vi "Dialog - Add Control.vi"(7 "Control":T3 {"Mech.Action" items=["Switch when Pressed", "Switch when Released", "Switch until Released", "Latch when Pressed", "Latch when Released", "Latch until Released"]; "Type" items=["Numeric", "Spin Control", "Vertical Slide", "Horizontal Slide", "Push Button", "Rocker", "Vert Rocker", "Horizontal Toggle Switch", "Vertical Toggle Switch", "Slide Switch", "Vertical Slide Switch", "OK Button", "Square Push Button", "Round Push Button", "Vertical Slide Switch2", "Square Push Button2", "Round Push Button2", "Horizontal Slide Switch2", "Round LED", "Square LED"]}, 11 "error in (no error)":errorcluster) -> (8 "Control Out":T3 {"Mech.Action" items=["Switch when Pressed", "Switch when Released", "Switch until Released", "Latch when Pressed", "Latch when Released", "Latch until Released"]; "Type" items=["Numeric", "Spin Control", "Vertical Slide", "Horizontal Slide", "Push Button", "Rocker", "Vert Rocker", "Horizontal Toggle Switch", "Vertical Toggle Switch", "Slide Switch", "Vertical Slide Switch", "OK Button", "Square Push Button", "Round Push Button", "Vertical Slide Switch2", "Square Push Button2", "Round Push Button2", "Horizontal Slide Switch2", "Round LED", "Square LED"]}, 10 "Cancelled":bool, 15 "error out":errorcluster)   [LabVIEW 2011]
uses:
  Default.ctl
panel:
  in  "Switched when pressed":T1 {"HSlide" scale=0.0..10.0; "VSlide" scale=0.0..10.0; "Box" min=0.0 max=10.0}
  in  "Switched when released":T1 {"HSlide" scale=0.0..10.0; "VSlide" scale=0.0..10.0}
  in  "Switched until released":T1 {"HSlide" scale=0.0..10.0; "VSlide" scale=0.0..10.0}
  in  "Colors":T2
  out "Test":bool
  in  "Action":u16(ring) items=["Switch when Pressed", "Switch when Released", "Switch until Released", "Latch when Pressed", "Latch when Released", "Latch until Released"]
  in  "Type":i32(ring) items=["Numeric", "Spin Control", "Vertical Slide", "Horizontal Slide", "Push Button", "Rocker", "Vert Rocker", "Horizontal Toggle Switch", "Vertical Toggle Switch", "Slide Switch", "Vertical Slide Switch", "OK Button", "Square Push Button", "Round Push Button", "Vertical Slide Switch2", "Square Push Button2", "Round Push Button2", "Horizontal Slide Switch2", "Round LED", "Square LED"]
  in  "Background":u32(colorbox)
  in  "Max":dbl
  in  "Min":dbl
  in  "Tip Strip":string
  in  "Label":string
  in  "Units":string
  in  "Name":string
  in  "Ok":bool
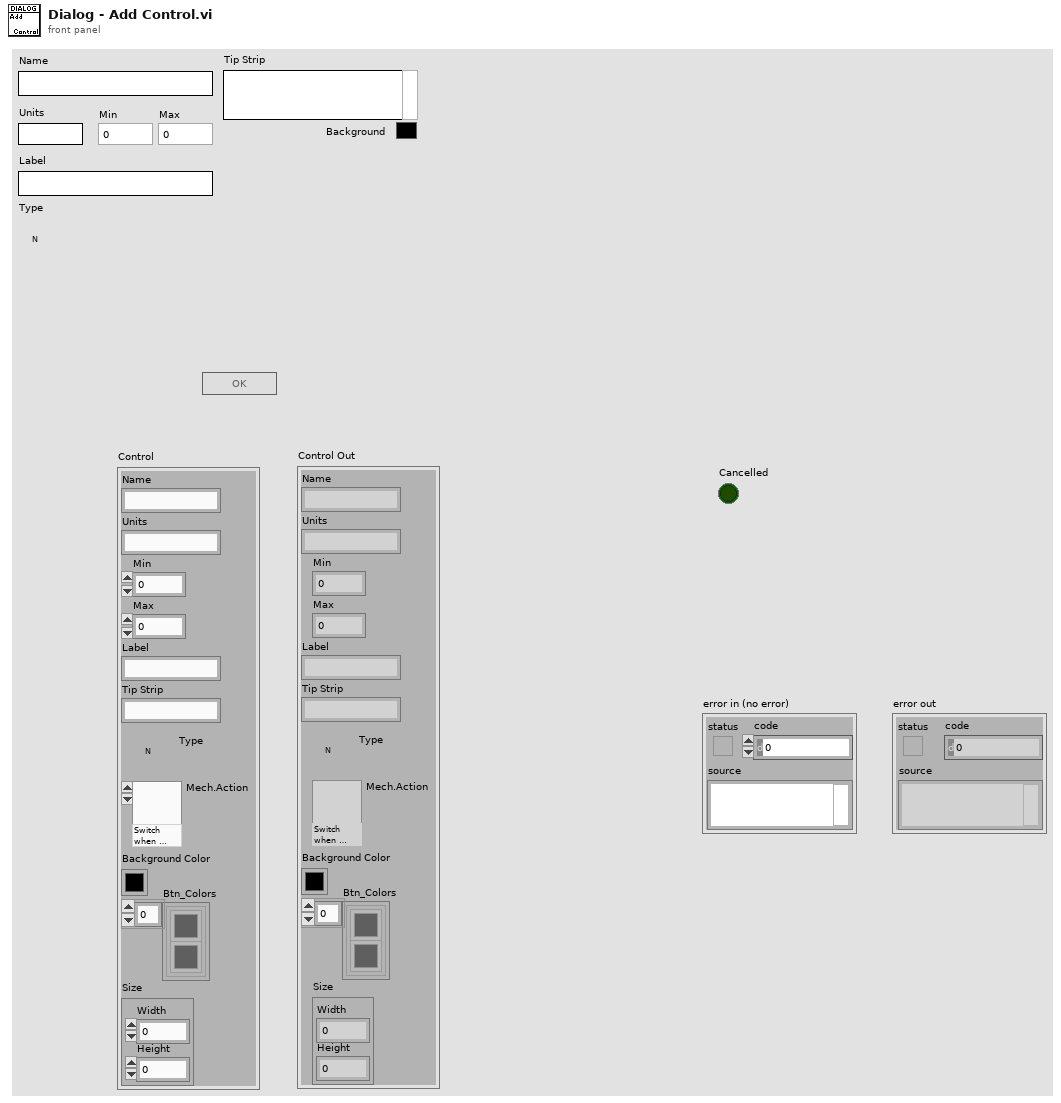
[diagram p1: front panel]
types:
  T1 = cluster{"Box":dbl[unit], "Spin":dbl[unit], "VSlide":dbl[unit], "HSlide":dbl[unit], "Push Button":bool, "HRocker":bool, "VRocker":bool, "HToggle":bool, "VToggle":bool, "HSlideSW":bool, "VSlideSW":bool, "System":bool, "Square Push Button":bool, "Round Push Button":bool, "VSlideSW2":bool, "Square Push Btn2":bool, "Round Push Btn2":bool, "HSlideSW2":bool, "Round LED":bool, "Square LED":bool}
  T2 = cluster{"F->T":cluster{"FG0":u32, "BG0":u32}, "F->T 2":cluster{"FG1":u32, "BG1":u32}, "F->T 3":cluster{"FG2":u32, "BG2":u32}, "F->T 4":cluster{"FG3":u32, "BG3":u32}}
  T3 = typedef "Default.ctl" = cluster{"Name":string, "Units":string, "Min":dbl, "Max":dbl, "Label":string, "Tip Strip":string, "Background Color":u32, "Type":i32, "Mech.Action":u16, "Btn_Colors ":cluster{"FG":u32, "BG":u32}[], "Size":cluster{"Width":u32, "Height":u32}}
  T4 = cluster{"Timeout":i32, "Control":T3, "PreVIEW":refnum<vi>}
  T5 = enum8{"Enabled", "Disabled", "Disabled and Grayed Out"}
  T6 = cluster{"Box":bool, "Spin":bool, "VSlide":bool, "HSlide":bool, "Push Button":bool, "HRocker":bool, "VRocker":bool, "HToggle":bool, "VToggle":bool, "HSlideSW":bool, "VSlideSW":bool, "System":bool, "Square Push Button":bool, "Round Push Button":bool, "VSlideSW2":bool, "Square Push Btn2":bool, "Round Push Btn2":bool, "HSlideSW2":bool, "Round LED":bool, "Square LED":bool}
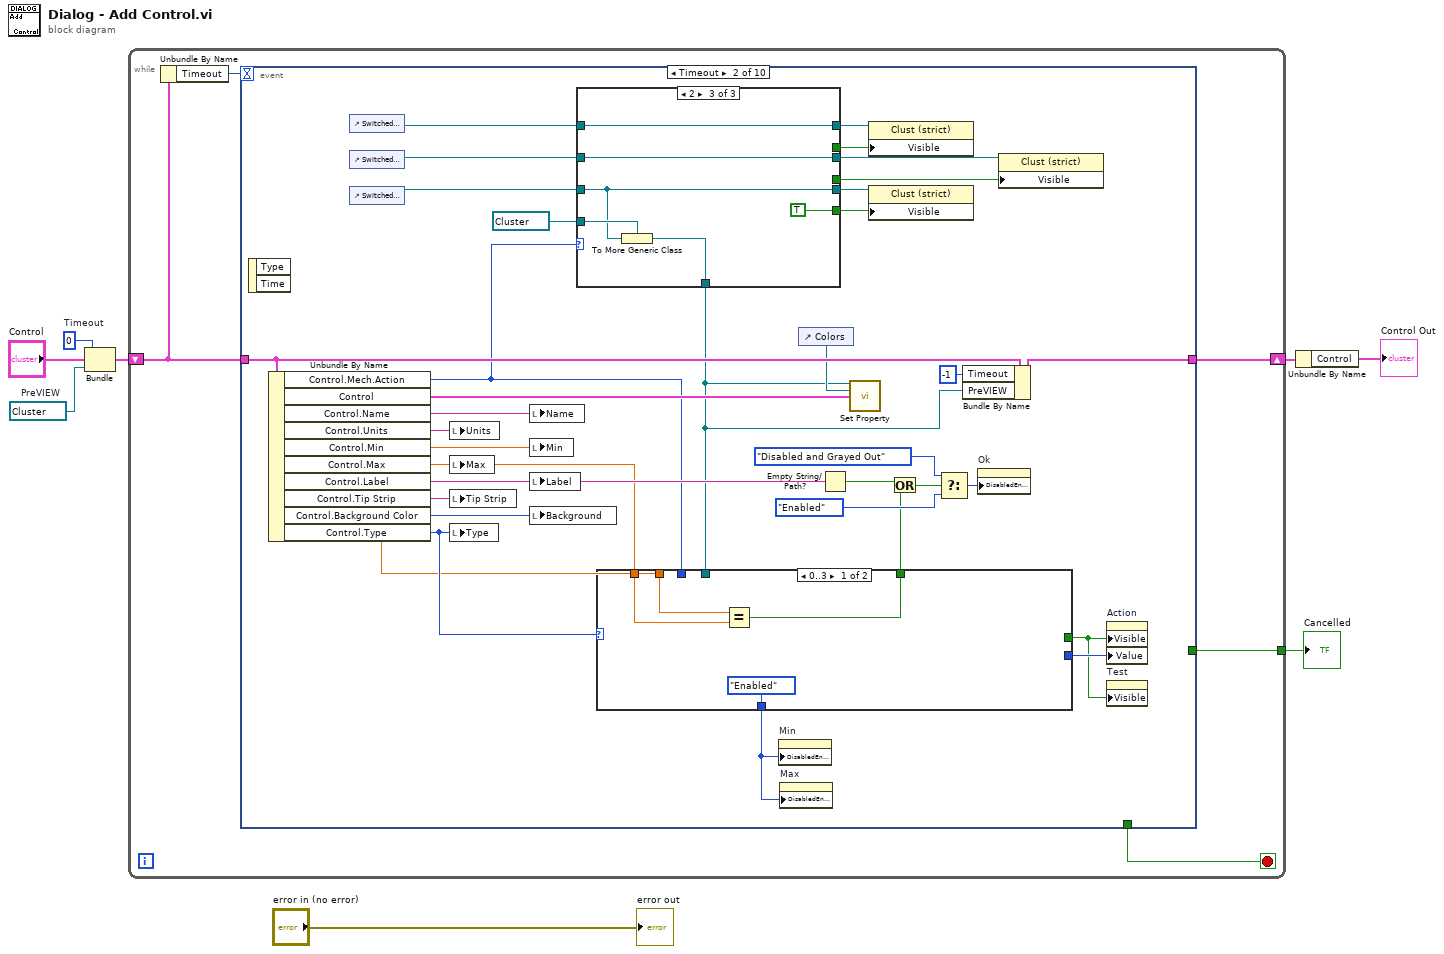
[diagram p0: block diagram]
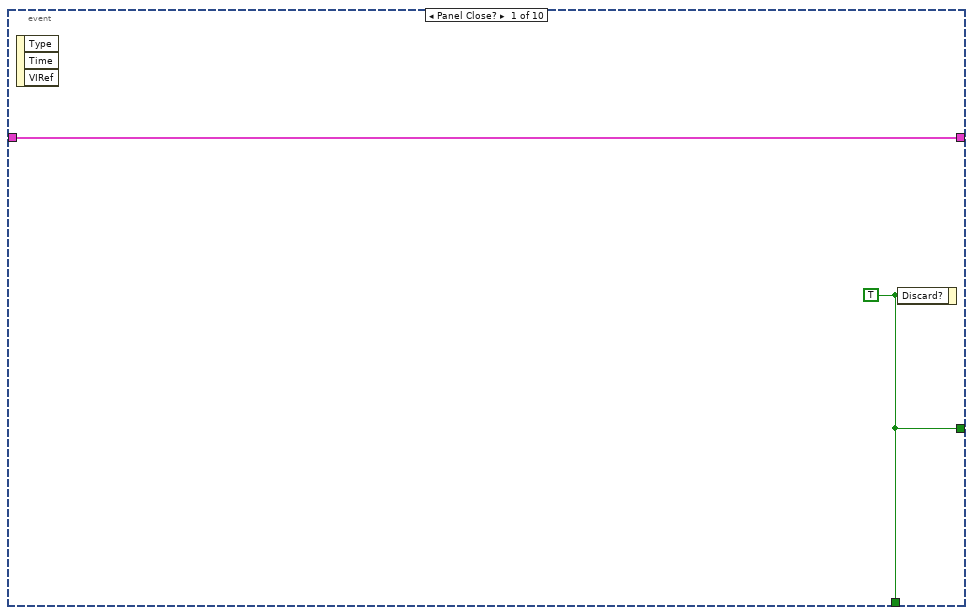
[diagram p2: hidden frame]
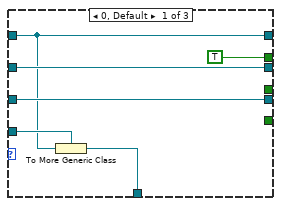
[diagram p3: hidden frame]
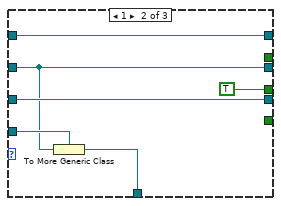
[diagram p4: hidden frame]
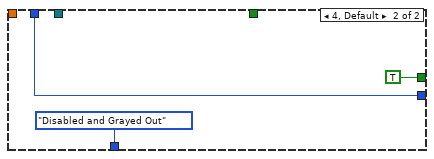
[diagram p5: hidden frame]
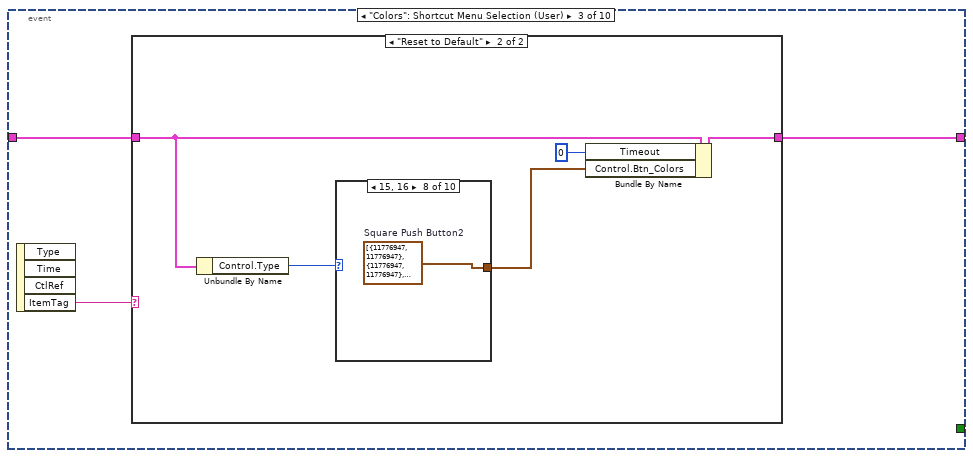
[diagram p6: hidden frame]
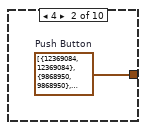
[diagram p9: hidden frame]
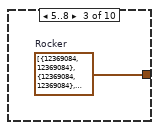
[diagram p10: hidden frame]
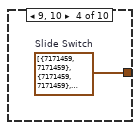
[diagram p11: hidden frame]
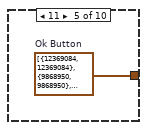
[diagram p12: hidden frame]
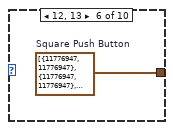
[diagram p13: hidden frame]
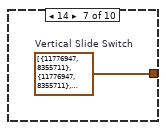
[diagram p14: hidden frame]
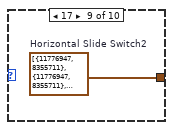
[diagram p15: hidden frame]
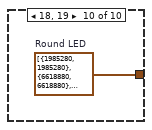
[diagram p16: hidden frame]
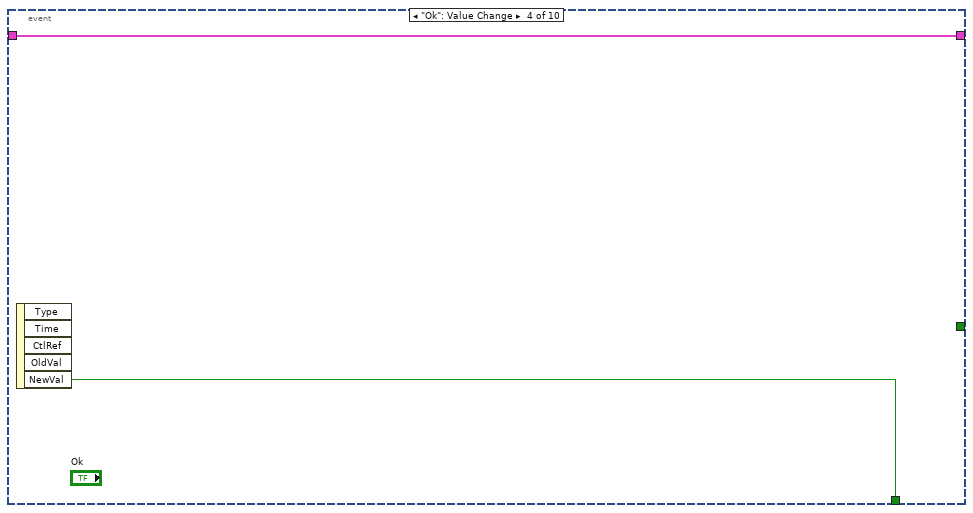
[diagram p17: hidden frame]
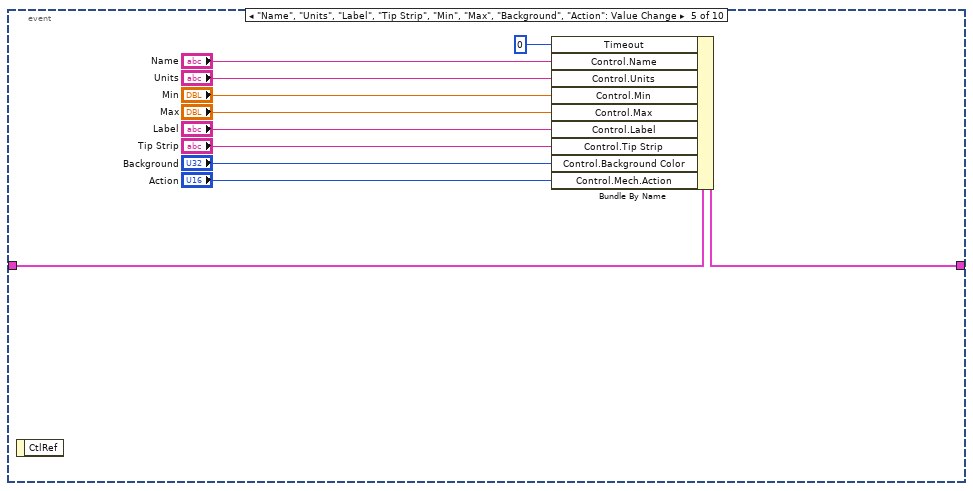
[diagram p18: hidden frame]
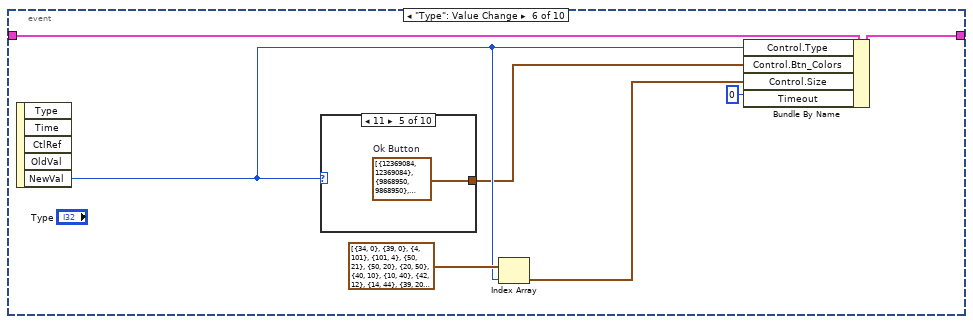
[diagram p19: hidden frame]
diagram:
  w1 = refnum<vi> refnum  # PreVIEW
  w6 = 0  # Timeout
  n1 = Bundle("Timeout"=w6, "Control"="Control", "PreVIEW"=w1) -> (w7:T4)  [unwired: 1 in]
  n2 = while {
    tunnel: [w12] -> w8
    shift-right: [w11] -> w4
    shift-left: w7 -> [w10]
    stop <- w13 stop-if-true
    n3 = Unbundle By Name(w10) -> ("Timeout"=w9:i32)
    n4 = event shown="[1] Timeout" {
      selector: _ -> [_ _ _ _ _ _ _ _ _ _]
      dyn-events: _ -> [_ _ _ _ _ _ _ _ _ _]
      timeout: w9 -> [_ _ _ _ _ _ _ _ _ _]
      tunnel: [w15 _ _ w94 _ _ _ _ _ _] -> w13
      tunnel: [w15 _ _ _ _ _ _ _ _ _] -> w12
      tunnel: w10 -> [w14 w49 w75 w93 w105 w112 w132 w144 w234 w245]
      tunnel: [w14 w48 w76 w93 w104 w111 w131 w144 w234 w245] -> w11
      event Panel Close? {
        w15 = TRUE ("Discard?")
        n5 = event-data() -> ()  [unwired: 1 in, 3 out]
        n6 = event-data("Discard?"=w15) -> ()  [unwired: 1 in, 1 out]
      }
      event Timeout {
        n7 = event-data() -> ()  [unwired: 1 in, 2 out]
        n8 = Unbundle By Name(w49) -> ("Control.Mech.Action"=w26:u16, "Control"=w43:T3, "Control.Name"=w46:string, "Control.Units"=w45:string, "Control.Min"=w22:dbl, "Control.Max"=w21:dbl, "Control.Label"=w41:string, "Control.Tip Strip"=w44:string, "Control.Background Color"=w42:u32, "Control.Type"=w35:i32)
        n9 = control-ref of="Switched when pressed"() -> (w18:refnum<vi>)
        n10 = control-ref of="Switched when released"() -> (w17:refnum<vi>)
        n11 = control-ref of="Switched until released"() -> (w16:refnum<vi>)
        n12 = local write "Units"(w45) -> ()
        n13 = local write "Max"(w21) -> ()
        n14 = local write "Tip Strip"(w44) -> ()
        n15 = local write "Type"(w35) -> ()
        n16 = local write "Name"(w46) -> ()
        n17 = local write "Min"(w22) -> ()
        n18 = local write "Label"(w41) -> ()
        n19 = local write "Background"(w42) -> ()
        n20 = case shown="2" w26 {
          tunnel: [w50 w56 w62] -> w23
          tunnel: w18 -> [w51 w61 w67]
          tunnel: w17 -> [w55 w57 w66]
          tunnel: w16 -> [w54 w60 w63]
          tunnel: [w51 w61 w67] -> w33
          tunnel: [w55 w57 w66] -> w32
          tunnel: [w54 w60 w63] -> w31
          tunnel: [TRUE _ _] -> w30
          tunnel: [_ TRUE _] -> w29
          tunnel: [_ _ TRUE] -> w28
          tunnel: refnum<vi> refnum ("PreVIEW") -> [w52 w58 w64]
          frame 0, Default {
            n21 = To More Generic Class(target class=w52, reference=w51) -> (generic class reference=w50:refnum<vi>)
          }
          frame 1 {
            n22 = To More Generic Class(target class=w58, reference=w57) -> (generic class reference=w56:refnum<vi>)
          }
          frame 2 {
            n23 = To More Generic Class(target class=w64, reference=w63) -> (generic class reference=w62:refnum<vi>)
          }
        }
        n24 = case shown="0..3" w35 {
          tunnel: w23 -> [_ _]
          tunnel: [_ w72] -> w34
          tunnel: [_ TRUE] -> w25
          tunnel: [T5."Enabled" ("Disabled") T5."Disabled and Grayed Out" ("Disabled")] -> w27
          tunnel: w26 -> [_ w72]
          tunnel: w22 -> [w70 _]
          tunnel: w21 -> [w69 _]
          tunnel: [w68 _] -> w20
          frame 0..3 {
            n25 = Equal?(x=w70, y=w69) -> (x = y?=w68:bool)
          }
          frame 4, Default {
          }
        }
        n26 = property on="Min" class="DigNum (strict)"("DisabledEnum"=w27) -> ()  [unwired: 2 in, 2 out]
        n27 = property on="Max" class="DigNum (strict)"("DisabledEnum"=w27) -> ()  [unwired: 2 in, 2 out]
        n28 = control-ref of="Colors"() -> (w24:refnum<vi>)
        n29 = Empty String/Path?(string/path=w41) -> (empty?=w39:bool)
        n30 = call "Set Property.vi"("Refnum"=w23, "Colors"=w24, "Property"=w43) -> ()  [unwired: 12 in, 1 out]
        n31 = property class="Clust (strict)"(reference=w33, "Visible"=w30) -> ()  [unwired: 1 in, 2 out]
        n32 = property class="Clust (strict)"(reference=w31, "Visible"=w28) -> ()  [unwired: 1 in, 2 out]
        n33 = Or(x=w39, y=w20) -> (x .or. y?=w36:bool)
        n34 = Select(t=T5."Disabled and Grayed Out" ("Disabled"), s=w36, f=T5."Enabled" ("Disabled")) -> (s? t:f=w40:T5)
        n35 = Bundle By Name(cluster=w49, "Timeout"=-1, "PreVIEW"=w23) -> (w48:T4)
        n36 = property on="Ok" class="Bool"("DisabledEnum"=w40) -> ()  [unwired: 2 in, 2 out]
        n37 = property class="Clust (strict)"(reference=w32, "Visible"=w29) -> ()  [unwired: 1 in, 2 out]
        n38 = property on="Action" class="Ring (strict)"("Visible"=w25, "Value"=w34) -> ()  [unwired: 2 in, 2 out]
        n39 = property on="Test" class="Bool (strict)"("Visible"=w25) -> ()  [unwired: 2 in, 2 out]
      }
      event "Colors": Shortcut Menu Selection (User) {
        n40 = event-data() -> ("ItemTag"=w77:string)  [unwired: 1 in, 3 out]
        n41 = case shown="\"Reset to Default\"" w77 {
          tunnel: [w78 w83] -> w76
          tunnel: w75 -> [w78 w80]
          frame "False", Default {
          }
          frame "Reset to Default" {
            n42 = Unbundle By Name(w80) -> ("Control.Type"=w79:i32)
            n43 = case shown="15, 16" w79 {
              tunnel: [_ w84 w85 w86 w87 w88 w89 w90 w91 w92] -> w81
              frame 0, Default {
              }
              frame 4 {
                w84 = cluster{u32, u32}[] [{12369084, 12369084}, {9868950, 9868950}, {12369084, 12369084}, {9868950, 9868950}]  # Push Button
              }
              frame 5..8 {
                w85 = cluster{u32, u32}[] [{12369084, 12369084}, {12369084, 12369084}, {12369084, 12369084}, {12369084, 12369084}]  # Rocker
              }
              frame 9, 10 {
                w86 = cluster{u32, u32}[] [{7171459, 7171459}, {7171459, 7171459}, {7171459, 7171459}, {7171459, 7171459}]  # Slide Switch
              }
              frame 11 {
                w87 = cluster{u32, u32}[] [{12369084, 12369084}, {9868950, 9868950}, {12369084, 12369084}, {9868950, 9868950}]  # Ok Button
              }
              frame 12, 13 {
                w88 = cluster{u32, u32}[] [{11776947, 11776947}, {11776947, 11776947}, {11776947, 11776947}, {11776947, 11776947}]  # Square Push Button
              }
              frame 14 {
                w89 = cluster{u32, u32}[] [{11776947, 8355711}, {11776947, 8355711}, {8355711, 8355711}, {8355711, 8355711}]  # Vertical Slide Switch
              }
              frame 15, 16 {
                w90 = cluster{u32, u32}[] [{11776947, 11776947}, {11776947, 11776947}, {11776947, 11776947}, {11776947, 11776947}]  # Square Push Button2
              }
              frame 17 {
                w91 = cluster{u32, u32}[] [{11776947, 8355711}, {11776947, 8355711}, {8355711, 8355711}, {8355711, 8355711}]  # Horizontal Slide Switch2
              }
              frame 18, 19 {
                w92 = cluster{u32, u32}[] [{1985280, 1985280}, {6618880, 6618880}, {1985280, 1985280}, {6618880, 6618880}]  # Round LED
              }
            }
            n44 = Bundle By Name(cluster=w80, "Timeout"=0, "Control.Btn_Colors"=w81) -> (w83:T4)
          }
        }
      }
      event "Ok": Value Change {
        n45 = event-data() -> ("NewVal"=w94:bool)  [unwired: 1 in, 4 out]
      }
      event "Name", "Units", "Label", "Tip Strip", "Min", "Max", "Background", "Action": Value Change {
        n46 = event-data() -> ()  [unwired: 1 in, 1 out]
        n47 = Bundle By Name(cluster=w105, "Timeout"=0, "Control.Name"="Name", "Control.Units"="Units", "Control.Min"="Min", "Control.Max"="Max", "Control.Label"="Label", "Control.Tip Strip"="Tip Strip", "Control.Background Color"="Background", "Control.Mech.Action"="Action") -> (w104:T4)
      }
      event "Type": Value Change {
        n48 = event-data() -> ("NewVal"=w108:i32)  [unwired: 1 in, 4 out]
        n49 = case shown="11" w108 {
          tunnel: [_ w113 w114 w115 w116 w117 w118 w119 w120 w121] -> w106
          frame 0, Default {
          }
          frame 4 {
            w113 = cluster{u32, u32}[] [{12369084, 12369084}, {9868950, 9868950}, {12369084, 12369084}, {9868950, 9868950}]  # Push Button
          }
          frame 5..8 {
            w114 = cluster{u32, u32}[] [{12369084, 12369084}, {12369084, 12369084}, {12369084, 12369084}, {12369084, 12369084}]  # Rocker
          }
          frame 9, 10 {
            w115 = cluster{u32, u32}[] [{7171459, 7171459}, {7171459, 7171459}, {7171459, 7171459}, {7171459, 7171459}]  # Slide Switch
          }
          frame 11 {
            w116 = cluster{u32, u32}[] [{12369084, 12369084}, {9868950, 9868950}, {12369084, 12369084}, {9868950, 9868950}]  # Ok Button
          }
          frame 12, 13 {
            w117 = cluster{u32, u32}[] [{11776947, 11776947}, {11776947, 11776947}, {11776947, 11776947}, {11776947, 11776947}]  # Square Push Button
          }
          frame 14 {
            w118 = cluster{u32, u32}[] [{11776947, 8355711}, {11776947, 8355711}, {8355711, 8355711}, {8355711, 8355711}]  # Vertical Slide Switch
          }
          frame 15, 16 {
            w119 = cluster{u32, u32}[] [{11776947, 11776947}, {11776947, 11776947}, {11776947, 11776947}, {11776947, 11776947}]  # Square Push Button2
          }
          frame 17 {
            w120 = cluster{u32, u32}[] [{11776947, 8355711}, {11776947, 8355711}, {8355711, 8355711}, {8355711, 8355711}]  # Horizontal Slide Switch2
          }
          frame 18, 19 {
            w121 = cluster{u32, u32}[] [{1985280, 1985280}, {6618880, 6618880}, {1985280, 1985280}, {6618880, 6618880}]  # Round LED
          }
        }
        n50 = Index Array(array=cluster{"Width":u32, "Height":u32}[] [{"Width"=34, "Height"=0}, {"Width"=39, "Height"=0}, {"Width"=4, "Height"=101}, {"Width"=101, "Height"=4}, {"Width"=50, "Height"=21}, {"Width"=50, "Height"=20}, {"Width"=20, "Height"=50}, {"Width"=40, "Height"=10}, {"Width"=10, "Height"=40}, {"Width"=42, "Height"=12}, {"Width"=14, "Height"=44}, {"Width"=39, "Height"=20}, {"Width"=30, "Height"=30}, {"Width"=30, "Height"=30}, {"Width"=19, "Height"=30}, {"Width"=27, "Height"=30}, {"Width"=27, "Height"=30}, {"Width"=30, "Height"=19}, {"Width"=17, "Height"=17}, {"Width"=24, "Height"=8}] ("Original Sizes"), index=w108) -> (element=w107:cluster{"Width":u32, "Height":u32})
        n51 = Bundle By Name(cluster=w112, "Control.Type"=w108, "Control.Btn_Colors"=w106, "Control.Size"=w107, "Timeout"=0) -> (w111:T4)
      }
      event "Colors": Value Change {
        n52 = event-data() -> ("CtlRef"=w126:refnum<vi>)  [unwired: 1 in]
        n53 = property class="Clust (strict)"(reference=w126) -> ("Controls[]"=w124:refnum<vi>[])  [unwired: 1 in, 2 out]
        n54 = Cluster To Array(cluster="Colors") -> (array=w128:cluster{"FG3":u32, "BG3":u32}[])
        n55 = for {
          tunnel: w124 -> [w137] mode=indexing
          tunnel: [w133] -> w123
          i -> [w133]
          stop <- w134 stop-if-true
          n56 = property class="Ctl"(reference=w137) -> ("DisabledEnum"=w136:T5)  [unwired: 1 in, 2 out]
          n57 = Equal?(x=w136, y=T5."Disabled and Grayed Out") -> (x = y?=w134:bool)
        }
        n58 = Increment(x=w123) -> (x+1=w122:i32)
        n59 = Array Subset(array=w128, index=0, length=w122) -> (w127:cluster{"FG3":u32, "BG3":u32}[])
        n60 = Bundle By Name(cluster=w132, "Timeout"=0, "Control.Btn_Colors"=w127) -> (w131:T4)
      }
      event "Colors.F->T.FG0", "Colors.F->T.BG0", "Colors.F->T 2.FG1", "Colors.F->T 2.BG1", "Colors.F->T 3.FG2", "Colors.F->T 3.BG2", "Colors.F->T 4.FG3", "Colors.F->T 4.BG3": Mouse Enter {
        n61 = event-data() -> ("CtlRef"=w141:refnum<vi>)  [unwired: 1 in]
        n62 = Unbundle By Name(w144) -> ("Control.Btn_Colors"=w138:cluster{"FG":u32, "BG":u32}[], "PreVIEW"=w143:refnum<vi>)
        n63 = property class="Clust"(reference=w143) -> ("Controls[]"=w142:refnum<vi>[])  [unwired: 1 in, 2 out]
        n64 = property class="ColBox"(reference=w141) -> ("Label.Text"=w140:string)  [unwired: 1 in, 2 out]
        n65 = for {
          tunnel: w142 -> [w227] mode=indexing
          tunnel: [w225] -> w139
          stop <- w226 stop-if-true
          n66 = property class="Ctl"(reference=w227) -> (reference out=w225:refnum<vi>, "Visible"=w226:bool)  [unwired: 1 in, 1 out]
        }
        n67 = case shown="\"FG0\"" w140 {
          tunnel: w139 -> [_ w154 w164 w174 w184 w194 w204 w214 w224]
          tunnel: w138 -> [_ w150 w160 w170 w180 w190 w200 w210 w220]
          frame "False", Default {
          }
          frame "FG0" {
            w149 = 0 ("index")
            w153 = refnum<vi> refnum  # Boolean
            n68 = Index Array(array=w150, index=w149) -> (element=w147:cluster{"FG":u32, "BG":u32})
            n69 = To More Specific Class(target class=w153, reference=w154) -> (specific class reference=w152:refnum<vi>)  [unwired: 1 in, 1 out]
            n70 = Unbundle(w147) -> ("FG"=w146:u32)  [unwired: 1 out]
            n71 = call <vilib>:"Hilite Color.vi"("Color In"=w146) -> ("Shadow"=w145:u32)  [unwired: 1 in, 1 out]
            n72 = Bundle(cluster=w147, "FG"=w145) -> (w148:cluster{"FG":u32, "BG":u32})  [unwired: 1 in]
            n73 = Replace Array Subset(array=w150, new element=w148, index=w149) -> (w151:cluster{"FG":u32, "BG":u32}[])
            n74 = property class="Bool"(reference=w152, "Colors [4]"=w151) -> ()  [unwired: 1 in, 2 out]
          }
          frame "FG1" {
            w159 = 1 ("index")
            w163 = refnum<vi> refnum  # Boolean
            n75 = Index Array(array=w160, index=w159) -> (element=w157:cluster{"FG":u32, "BG":u32})
            n76 = To More Specific Class(target class=w163, reference=w164) -> (specific class reference=w162:refnum<vi>)  [unwired: 1 in, 1 out]
            n77 = Unbundle(w157) -> ("FG"=w156:u32)  [unwired: 1 out]
            n78 = call <vilib>:"Hilite Color.vi"("Color In"=w156) -> ("Shadow"=w155:u32)  [unwired: 1 in, 1 out]
            n79 = Bundle(cluster=w157, "FG"=w155) -> (w158:cluster{"FG":u32, "BG":u32})  [unwired: 1 in]
            n80 = Replace Array Subset(array=w160, new element=w158, index=w159) -> (w161:cluster{"FG":u32, "BG":u32}[])
            n81 = property class="Bool"(reference=w162, "Colors [4]"=w161) -> ()  [unwired: 1 in, 2 out]
          }
          frame "FG2" {
            w169 = 2 ("index")
            w173 = refnum<vi> refnum  # Boolean
            n82 = Index Array(array=w170, index=w169) -> (element=w167:cluster{"FG":u32, "BG":u32})
            n83 = To More Specific Class(target class=w173, reference=w174) -> (specific class reference=w172:refnum<vi>)  [unwired: 1 in, 1 out]
            n84 = Unbundle(w167) -> ("FG"=w166:u32)  [unwired: 1 out]
            n85 = call <vilib>:"Hilite Color.vi"("Color In"=w166) -> ("Shadow"=w165:u32)  [unwired: 1 in, 1 out]
            n86 = Bundle(cluster=w167, "FG"=w165) -> (w168:cluster{"FG":u32, "BG":u32})  [unwired: 1 in]
            n87 = Replace Array Subset(array=w170, new element=w168, index=w169) -> (w171:cluster{"FG":u32, "BG":u32}[])
            n88 = property class="Bool"(reference=w172, "Colors [4]"=w171) -> ()  [unwired: 1 in, 2 out]
          }
          frame "FG3" {
            w179 = 3 ("index")
            w183 = refnum<vi> refnum  # Boolean
            n89 = Index Array(array=w180, index=w179) -> (element=w177:cluster{"FG":u32, "BG":u32})
            n90 = To More Specific Class(target class=w183, reference=w184) -> (specific class reference=w182:refnum<vi>)  [unwired: 1 in, 1 out]
            n91 = Unbundle(w177) -> ("FG"=w176:u32)  [unwired: 1 out]
            n92 = call <vilib>:"Hilite Color.vi"("Color In"=w176) -> ("Shadow"=w175:u32)  [unwired: 1 in, 1 out]
            n93 = Bundle(cluster=w177, "FG"=w175) -> (w178:cluster{"FG":u32, "BG":u32})  [unwired: 1 in]
            n94 = Replace Array Subset(array=w180, new element=w178, index=w179) -> (w181:cluster{"FG":u32, "BG":u32}[])
            n95 = property class="Bool"(reference=w182, "Colors [4]"=w181) -> ()  [unwired: 1 in, 2 out]
          }
          frame "BG0" {
            w189 = 0 ("index")
            w193 = refnum<vi> refnum  # Boolean
            n96 = Index Array(array=w190, index=w189) -> (element=w187:cluster{"FG":u32, "BG":u32})
            n97 = To More Specific Class(target class=w193, reference=w194) -> (specific class reference=w192:refnum<vi>)  [unwired: 1 in, 1 out]
            n98 = Unbundle(w187) -> ("BG"=w186:u32)  [unwired: 1 out]
            n99 = call <vilib>:"Hilite Color.vi"("Color In"=w186) -> ("Shadow"=w185:u32)  [unwired: 1 in, 1 out]
            n100 = Bundle(cluster=w187, "BG"=w185) -> (w188:cluster{"FG":u32, "BG":u32})  [unwired: 1 in]
            n101 = Replace Array Subset(array=w190, new element=w188, index=w189) -> (w191:cluster{"FG":u32, "BG":u32}[])
            n102 = property class="Bool"(reference=w192, "Colors [4]"=w191) -> ()  [unwired: 1 in, 2 out]
          }
          frame "BG1" {
            w199 = 1 ("index")
            w203 = refnum<vi> refnum  # Boolean
            n103 = Index Array(array=w200, index=w199) -> (element=w197:cluster{"FG":u32, "BG":u32})
            n104 = To More Specific Class(target class=w203, reference=w204) -> (specific class reference=w202:refnum<vi>)  [unwired: 1 in, 1 out]
            n105 = Unbundle(w197) -> ("BG"=w196:u32)  [unwired: 1 out]
            n106 = call <vilib>:"Hilite Color.vi"("Color In"=w196) -> ("Shadow"=w195:u32)  [unwired: 1 in, 1 out]
            n107 = Bundle(cluster=w197, "BG"=w195) -> (w198:cluster{"FG":u32, "BG":u32})  [unwired: 1 in]
            n108 = Replace Array Subset(array=w200, new element=w198, index=w199) -> (w201:cluster{"FG":u32, "BG":u32}[])
            n109 = property class="Bool"(reference=w202, "Colors [4]"=w201) -> ()  [unwired: 1 in, 2 out]
          }
          frame "BG2" {
            w209 = 2 ("index")
            w213 = refnum<vi> refnum  # Boolean
            n110 = Index Array(array=w210, index=w209) -> (element=w207:cluster{"FG":u32, "BG":u32})
            n111 = To More Specific Class(target class=w213, reference=w214) -> (specific class reference=w212:refnum<vi>)  [unwired: 1 in, 1 out]
            n112 = Unbundle(w207) -> ("BG"=w206:u32)  [unwired: 1 out]
            n113 = call <vilib>:"Hilite Color.vi"("Color In"=w206) -> ("Shadow"=w205:u32)  [unwired: 1 in, 1 out]
            n114 = Bundle(cluster=w207, "BG"=w205) -> (w208:cluster{"FG":u32, "BG":u32})  [unwired: 1 in]
            n115 = Replace Array Subset(array=w210, new element=w208, index=w209) -> (w211:cluster{"FG":u32, "BG":u32}[])
            n116 = property class="Bool"(reference=w212, "Colors [4]"=w211) -> ()  [unwired: 1 in, 2 out]
          }
          frame "BG3" {
            w219 = 3 ("index")
            w223 = refnum<vi> refnum  # Boolean
            n117 = Index Array(array=w220, index=w219) -> (element=w217:cluster{"FG":u32, "BG":u32})
            n118 = To More Specific Class(target class=w223, reference=w224) -> (specific class reference=w222:refnum<vi>)  [unwired: 1 in, 1 out]
            n119 = Unbundle(w217) -> ("BG"=w216:u32)  [unwired: 1 out]
            n120 = call <vilib>:"Hilite Color.vi"("Color In"=w216) -> ("Shadow"=w215:u32)  [unwired: 1 in, 1 out]
            n121 = Bundle(cluster=w217, "BG"=w215) -> (w218:cluster{"FG":u32, "BG":u32})  [unwired: 1 in]
            n122 = Replace Array Subset(array=w220, new element=w218, index=w219) -> (w221:cluster{"FG":u32, "BG":u32}[])
            n123 = property class="Bool"(reference=w222, "Colors [4]"=w221) -> ()  [unwired: 1 in, 2 out]
          }
        }
      }
      event "Colors.F->T.FG0", "Colors.F->T.BG0", "Colors.F->T 2.FG1", "Colors.F->T 2.BG1", "Colors.F->T 3.FG2", "Colors.F->T 3.BG2", "Colors.F->T 4.FG3", "Colors.F->T 4.BG3": Mouse Leave {
        w229 = refnum<vi> refnum  # Boolean
        n124 = event-data() -> ()  [unwired: 1 in, 1 out]
        n125 = Unbundle By Name(w234) -> ("Control.Btn_Colors"=w230:cluster{"FG":u32, "BG":u32}[], "PreVIEW"=w233:refnum<vi>)
        n126 = property class="Clust"(reference=w233) -> ("Controls[]"=w232:refnum<vi>[])  [unwired: 1 in, 2 out]
        n127 = for {
          tunnel: w232 -> [w237] mode=indexing
          tunnel: [w235] -> w231
          stop <- w236 stop-if-true
          n128 = property class="Ctl"(reference=w237) -> (reference out=w235:refnum<vi>, "Visible"=w236:bool)  [unwired: 1 in, 1 out]
        }
        n129 = To More Specific Class(target class=w229, reference=w231) -> (specific class reference=w228:refnum<vi>)  [unwired: 1 in, 1 out]
        n130 = property class="Bool"(reference=w228, "Colors [4]"=w230) -> ()  [unwired: 1 in, 2 out]
      }
      event "Switched until released", "Switched when released", "Switched when pressed": Value Change {
        n131 = event-data() -> ("OldVal"=w244:T1, "NewVal"=w239:T1)  [unwired: 1 in]
        n132 = Not Equal?(x=w244, y=w239) -> (x != y?=w243:T6)
        n133 = Cluster To Array(cluster=w243) -> (array=w242:bool[])
        n134 = Search 1D Array(1D array=w242, element=TRUE) -> (index of element=w240:i32)  [unwired: 1 in]
        n135 = case shown="19" w240 {
          tunnel: w239 -> [_ w247 w249 w251 w253 w255 w257 w259 w261 w263 w265 w267 w269 w271 w273 w275 w277]
          tunnel: [_ w246 w248 w250 w252 w254 w256 w258 w260 w262 w264 w266 w268 w270 w272 w274 w276] -> w238
          frame 0, Default {
          }
          frame 4 {
            n136 = Unbundle By Name(w247) -> ("Push Button"=w246:bool)
          }
          frame 5 {
            n137 = Unbundle By Name(w249) -> ("HRocker"=w248:bool)
          }
          frame 6 {
            n138 = Unbundle By Name(w251) -> ("VRocker"=w250:bool)
          }
          frame 7 {
            n139 = Unbundle By Name(w253) -> ("HToggle"=w252:bool)
          }
          frame 8 {
            n140 = Unbundle By Name(w255) -> ("VToggle"=w254:bool)
          }
          frame 9 {
            n141 = Unbundle By Name(w257) -> ("HSlideSW"=w256:bool)
          }
          frame 10 {
            n142 = Unbundle By Name(w259) -> ("VSlideSW"=w258:bool)
          }
          frame 11 {
            n143 = Unbundle By Name(w261) -> ("System"=w260:bool)
          }
          frame 12 {
            n144 = Unbundle By Name(w263) -> ("Square Push Button"=w262:bool)
          }
          frame 13 {
            n145 = Unbundle By Name(w265) -> ("Round Push Button"=w264:bool)
          }
          frame 14 {
            n146 = Unbundle By Name(w267) -> ("VSlideSW2"=w266:bool)
          }
          frame 15 {
            n147 = Unbundle By Name(w269) -> ("Square Push Btn2"=w268:bool)
          }
          frame 16 {
            n148 = Unbundle By Name(w271) -> ("Round Push Btn2"=w270:bool)
          }
          frame 17 {
            n149 = Unbundle By Name(w273) -> ("HSlideSW2"=w272:bool)
          }
          frame 18 {
            n150 = Unbundle By Name(w275) -> ("Round LED"=w274:bool)
          }
          frame 19 {
            n151 = Unbundle By Name(w277) -> ("Square LED"=w276:bool)
          }
        }
        "Test" <- w238
      }
    }
  }
  "Cancelled" <- w8
  n152 = Unbundle By Name(w4) -> ("Control"=→"Control Out":T3)
  "error out" <- "error in (no error)"
